vi "MCS_GetPosition.vi"(2 "error in (no error)":errorcluster, 3 "Channel Index In":u32, 4 "System Index In":u32) -> (0 "error out":errorcluster, 1 "Position (um)":dbl)   [LabVIEW 2010]
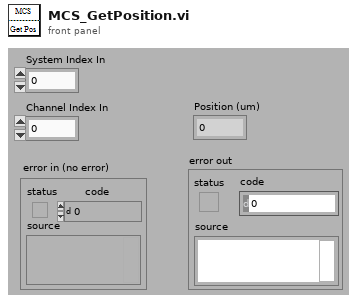
[diagram p1: front panel]
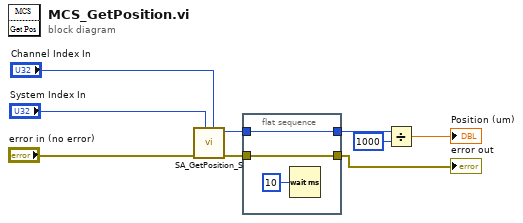
[diagram p0: block diagram]
diagram:
  n1 = call <vilib>:"SA_GetPosition_S.vi"("channelIndex"="Channel Index In", "systemIndex"="System Index In", "error in (no error)"="error in (no error)") -> ("error out"=w5:errorcluster, "position"=w6:i32)  [unwired: 7 in]
  n2 = flat-sequence {
    tunnel: [w11] -> w3
    tunnel: w6 -> [w11]
    tunnel: [w10] -> w4
    tunnel: w5 -> [w10]
    frame #0 {
      n3 = Wait (ms)(milliseconds to wait=u32 10) -> ()  [unwired: 1 out]
    }
  }
  n4 = Divide(x=w3, y=1000) -> (x/y=→"Position (um)":dbl)
  "error out" <- w4
